vi "Multiply Vector By Matrix.vi"(10 "Matrix in":sgl[][](array[numeric]), 11 "Vector 3D in":T1) -> (3 "Vector 3D out":T1)   [LabVIEW 2022 SP3, in "3D.lvlib"]
uses:
  3D.lvlib
  Vector 3D.ctl
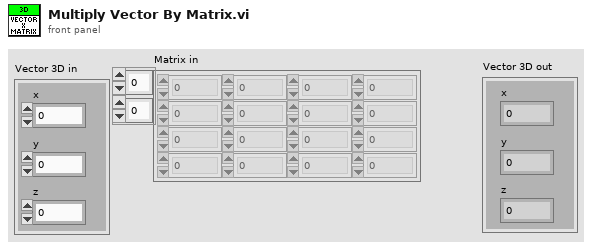
[diagram p1: front panel]
types:
  T1 = typedef "3D.lvlib/Vector 3D.ctl" = cluster{"x":sgl, "y":sgl, "z":sgl}
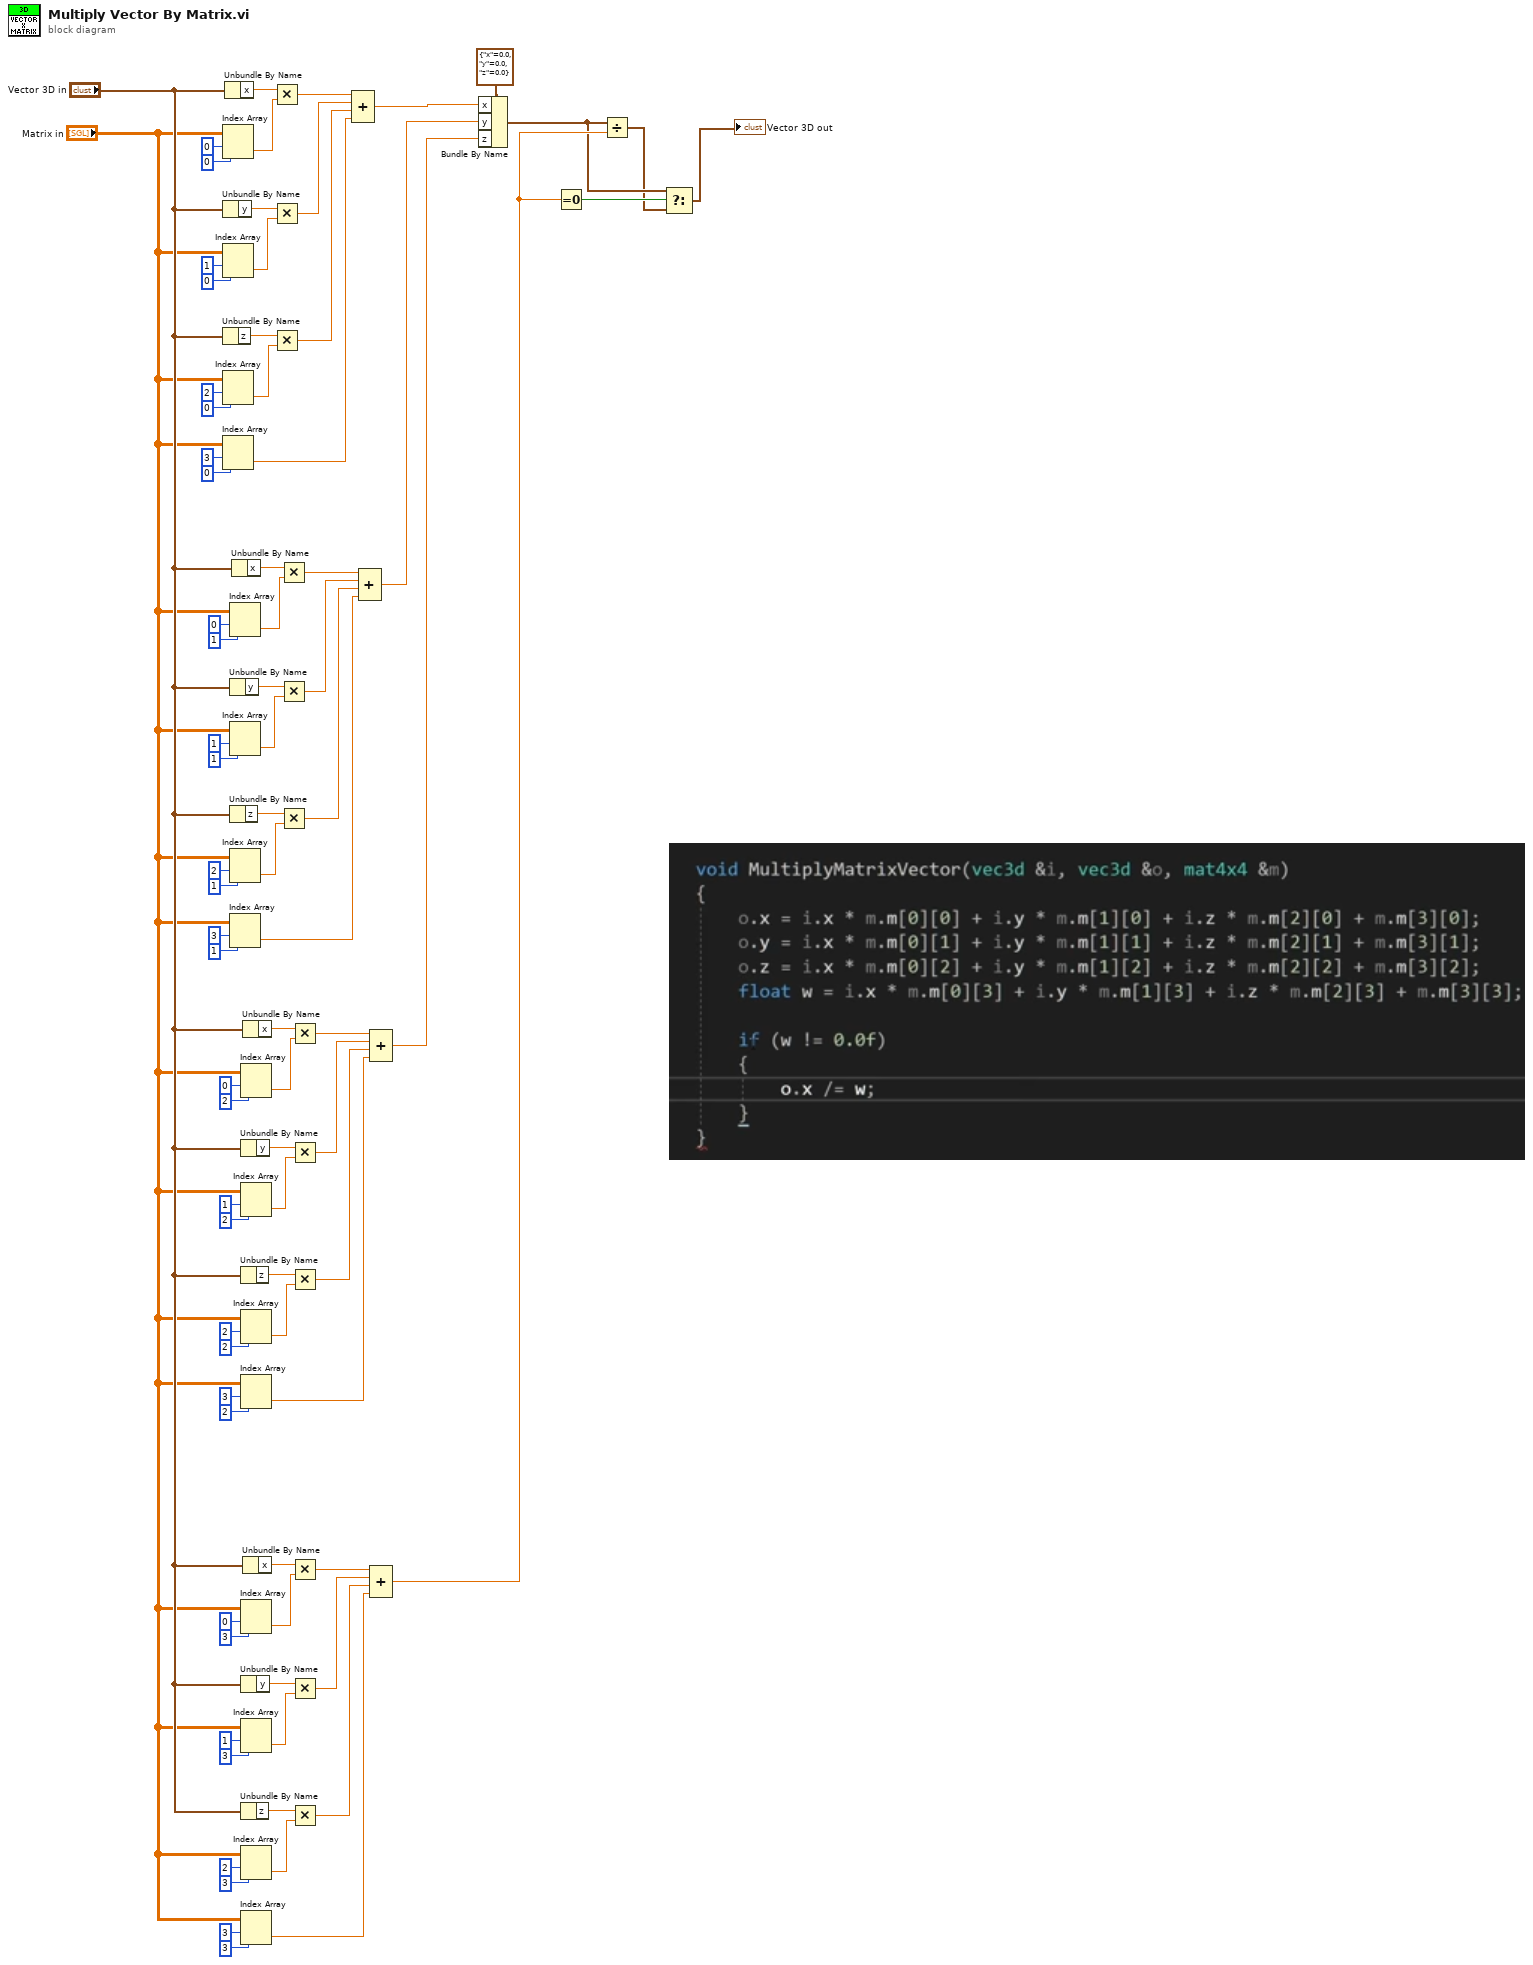
[diagram p0: block diagram]
diagram:
  n1 = Index Array(array="Matrix in", index (row)=0, index (col)=0 ("disabled index (col)")) -> (element=w79:sgl)
  n2 = Unbundle By Name("Vector 3D in") -> ("y"=w77:sgl)
  n3 = Index Array(array="Matrix in", index (row)=1, index (col)=0 ("disabled index (col)")) -> (element=w78:sgl)
  n4 = Unbundle By Name("Vector 3D in") -> ("z"=w72:sgl)
  n5 = Index Array(array="Matrix in", index (row)=2, index (col)=0 ("disabled index (col)")) -> (element=w71:sgl)
  n6 = Index Array(array="Matrix in", index (row)=3, index (col)=0 ("disabled index (col)")) -> (element=w65:sgl)
  n7 = Unbundle By Name("Vector 3D in") -> ("x"=w80:sgl)
  n8 = Index Array(array="Matrix in", index (row)=0, index (col)=1 ("disabled index (col)")) -> (element=w49:sgl)
  n9 = Unbundle By Name("Vector 3D in") -> ("y"=w51:sgl)
  n10 = Index Array(array="Matrix in", index (row)=1, index (col)=1 ("disabled index (col)")) -> (element=w50:sgl)
  n11 = Unbundle By Name("Vector 3D in") -> ("z"=w56:sgl)
  n12 = Index Array(array="Matrix in", index (row)=2, index (col)=1 ("disabled index (col)")) -> (element=w57:sgl)
  n13 = Index Array(array="Matrix in", index (row)=3, index (col)=1 ("disabled index (col)")) -> (element=w63:sgl)
  n14 = Unbundle By Name("Vector 3D in") -> ("x"=w48:sgl)
  n15 = Index Array(array="Matrix in", index (row)=0, index (col)=2 ("disabled index (col)")) -> (element=w41:sgl)
  n16 = Unbundle By Name("Vector 3D in") -> ("y"=w39:sgl)
  n17 = Index Array(array="Matrix in", index (row)=1, index (col)=2 ("disabled index (col)")) -> (element=w40:sgl)
  n18 = Unbundle By Name("Vector 3D in") -> ("z"=w34:sgl)
  n19 = Index Array(array="Matrix in", index (row)=2, index (col)=2 ("disabled index (col)")) -> (element=w33:sgl)
  n20 = Index Array(array="Matrix in", index (row)=3, index (col)=2 ("disabled index (col)")) -> (element=w27:sgl)
  n21 = Index Array(array="Matrix in", index (row)=0, index (col)=3 ("disabled index (col)")) -> (element=w11:sgl)
  n22 = Unbundle By Name("Vector 3D in") -> ("y"=w13:sgl)
  n23 = Index Array(array="Matrix in", index (row)=1, index (col)=3 ("disabled index (col)")) -> (element=w12:sgl)
  n24 = Unbundle By Name("Vector 3D in") -> ("z"=w18:sgl)
  n25 = Index Array(array="Matrix in", index (row)=2, index (col)=3 ("disabled index (col)")) -> (element=w19:sgl)
  n26 = Index Array(array="Matrix in", index (row)=3, index (col)=3 ("disabled index (col)")) -> (element=w25:sgl)
  n27 = Unbundle By Name("Vector 3D in") -> ("x"=w42:sgl)
  n28 = Unbundle By Name("Vector 3D in") -> ("x"=w10:sgl)
  n29 = Multiply(x=w80, y=w79) -> (x*y=w68:sgl)
  n30 = Multiply(x=w77, y=w78) -> (x*y=w67:sgl)
  n31 = Multiply(x=w72, y=w71) -> (x*y=w66:sgl)
  n32 = Multiply(x=w48, y=w49) -> (x*y=w60:sgl)
  n33 = Multiply(x=w51, y=w50) -> (x*y=w61:sgl)
  n34 = Multiply(x=w56, y=w57) -> (x*y=w62:sgl)
  n35 = Multiply(x=w42, y=w41) -> (x*y=w30:sgl)
  n36 = Multiply(x=w39, y=w40) -> (x*y=w29:sgl)
  n37 = Multiply(x=w34, y=w33) -> (x*y=w28:sgl)
  n38 = Multiply(x=w10, y=w11) -> (x*y=w22:sgl)
  n39 = Multiply(x=w13, y=w12) -> (x*y=w23:sgl)
  n40 = Multiply(x=w18, y=w19) -> (x*y=w24:sgl)
  n41 = Compound Arithmetic op=ADD(w68, w67, w66, w65) -> (w64:sgl)
  n42 = Compound Arithmetic op=ADD(w60, w61, w62, w63) -> (w45:sgl)
  n43 = Compound Arithmetic op=ADD(w30, w29, w28, w27) -> (w26:sgl)
  n44 = Compound Arithmetic op=ADD(w22, w23, w24, w25) -> (w5:sgl)
  n45 = Bundle By Name(cluster=T1 {"x"=0.0, "y"=0.0, "z"=0.0} ("Vector 3D in"), "x"=w64, "y"=w45, "z"=w26) -> (w3:T1)
  n46 = Equal To 0?(x=w5) -> (x = 0?=w4:bool)
  n47 = Divide(x=w3, y=w5) -> (x/y=w1:T1)
  n48 = Select(t=w3, s=w4, f=w1) -> (s? t:f=→"Vector 3D out":T1)
